vi "Open Statement.vi"(4 "error in (no error)":errorcluster, 7 "Connection Refnum":T1) -> (0 "error out":errorcluster, 3 "Statement Refnum":T2)   [LabVIEW 2011]
doc: "Etablit un lien de requête à destination des paramètres"
uses:
  SQL Controls/Statement Refnum.ctl
  SQL Controls/Connection Refnum.ctl
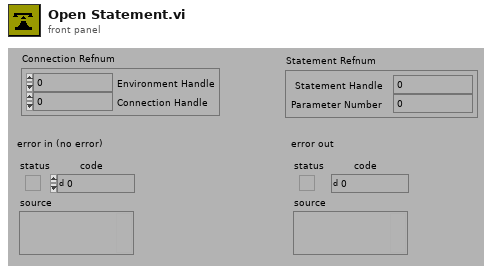
[diagram p1: front panel]
types:
  T1 = typedef "Connection Refnum.ctl" = cluster{"Environment Handle":i32, "Connection Handle":i32}
  T2 = typedef "Statement Refnum.ctl" = cluster{"Statement Handle":i32, "Parameter Number":u16}
  T3 = enum16{"NOPE", "SQL_HANDLE_ENV", "SQL_HANDLE_DBC", "SQL_HANDLE_STMT", "SQL_HANDLE_DESC"}
  T4 = cluster{"OutputHandle":i32, "Parameter Number":u16}
  T5 = cluster{"Statement Handle":i32, "Parameter Number":u16}
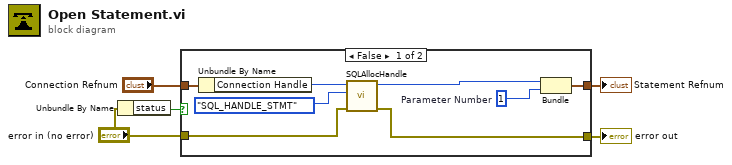
[diagram p0: block diagram]
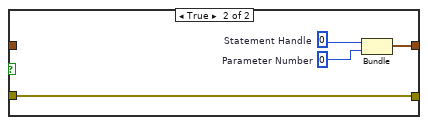
[diagram p2: hidden frame]
diagram:
  n1 = Unbundle By Name("error in (no error)") -> ("status"=w1:bool)
  n2 = case shown="False" w1 {
    tunnel: "Connection Refnum" -> [w12 _]
    tunnel: "error in (no error)" -> [w9 w17]
    tunnel: [w7 w15] -> w4
    tunnel: [w6 w17] -> w3
    frame False {
      w13 = u16 1  # Parameter Number
      n3 = Unbundle By Name(w12) -> ("Connection Handle"=w11:i32)
      n4 = call "SQLAllocHandle.vi"("error in (no error)"=w9, "HandleType"=T3."SQL_HANDLE_STMT", "InputHandle"=w11) -> ("error out"=w6:errorcluster, "OutputHandle"=w8:i32)  [unwired: 2 in, 1 out]
      n5 = Bundle("OutputHandle"=w8, "Parameter Number"=w13) -> (w7:T4)  [unwired: 1 out]
    }
    frame True {
      w16 = u16 0  # Parameter Number
      w14 = 0  # Statement Handle
      n6 = Bundle("Statement Handle"=w14, "Parameter Number"=w16) -> (w15:T5)  [unwired: 1 out]
    }
  }
  "Statement Refnum" <- w4
  "error out" <- w3
